vi "Set Property.vi"(8 "error in (no error)":errorcluster, 9 "Value":dbl, 10 "Property":string, 11 "SAM in":refnum<class "SAM.lvclass">) -> (0 "error out":errorcluster, 3 "SAM out":refnum<class "SAM.lvclass">)   [LabVIEW 2020, in "SAM.lvclass"]
uses:
  SAM.lvclass
  D:/Experiment VIs/Signal Synthesis VIs/4th Generation/Classes/Modulations/AM/AM.lvclass
  SAM.lvclass/SAM.ctl
  AM/AM.lvclass/AM.ctl
  AM/Write Depth (0-1).vi
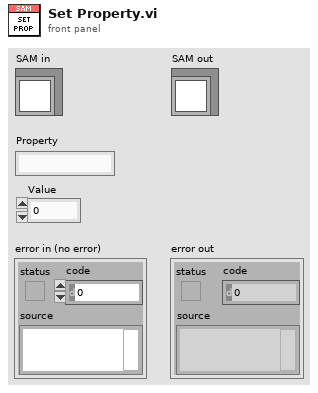
[diagram p1: front panel]
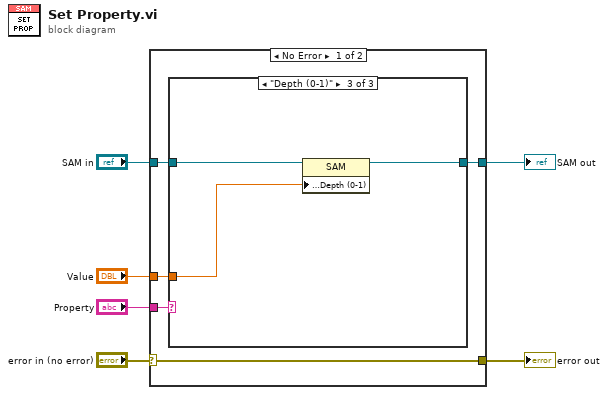
[diagram p0: block diagram]
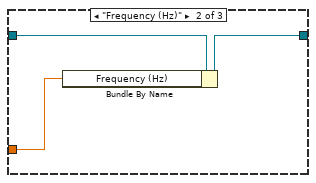
[diagram p3: hidden frame]
diagram:
  n1 = case shown="No Error" "error in (no error)" {
    selector: "error in (no error)" -> [w7 w19]
    tunnel: [w7 w19] -> w4
    tunnel: "Property" -> [w11 _]
    tunnel: "SAM in" -> [w10 w20]
    tunnel: "Value" -> [w9 _]
    tunnel: [w8 w20] -> w5
    frame No Error {
      n2 = case shown="\"Depth (0-1)\"" w11 {
        tunnel: w10 -> [w12 w15 w18]
        tunnel: w9 -> [_ w14 w16]
        tunnel: [w12 w13 w17] -> w8
        frame "", Default {
        }
        frame "Frequency (Hz)" {
          n3 = Bundle By Name(cluster=w15, "Frequency (Hz)"=w14) -> (w13:refnum<class "SAM.lvclass">)
        }
        frame "Depth (0-1)" {
          n4 = property class="SAM"(reference=w18, "Accessors:Depth (0-1)"=w16) -> (reference out=w17:refnum<class "SAM.lvclass">)  [unwired: 1 in, 1 out]
        }
      }
    }
    frame Error {
    }
  }
  "error out" <- w4
  "SAM out" <- w5
